vi "SDCP SMF Rx Logger - Base (version 1.1).vi"() -> ()   [LabVIEW 2020]
uses:
  Typedefs/SDCP - Serial Port Control - Commands.ctl
  Typedefs/SDCP SMF logger - SMF with timestamp.ctl
panel:
  out "error out":errorcluster
  in  "error in (no error)":errorcluster
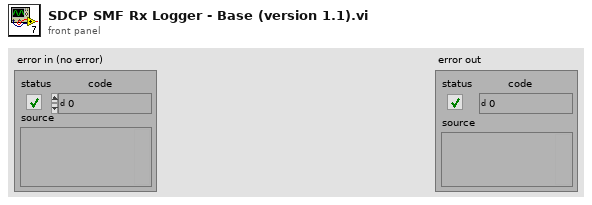
[diagram p1: front panel]
types:
  T1 = enum16{"Initialize", "Read", "Write", "Deinitialize"}
  T2 = typedef "SDCP SMF logger - SMF with timestamp.ctl" = cluster{"Bytes":u8[], "Checksum":bool, "Time (ms)":u32, "Tx/Rx":string}
  T3 = typedef "SDCP - Serial Port Control - Commands.ctl" = enum16{"Open", "Read", "Write", "Get instance", "Close"}
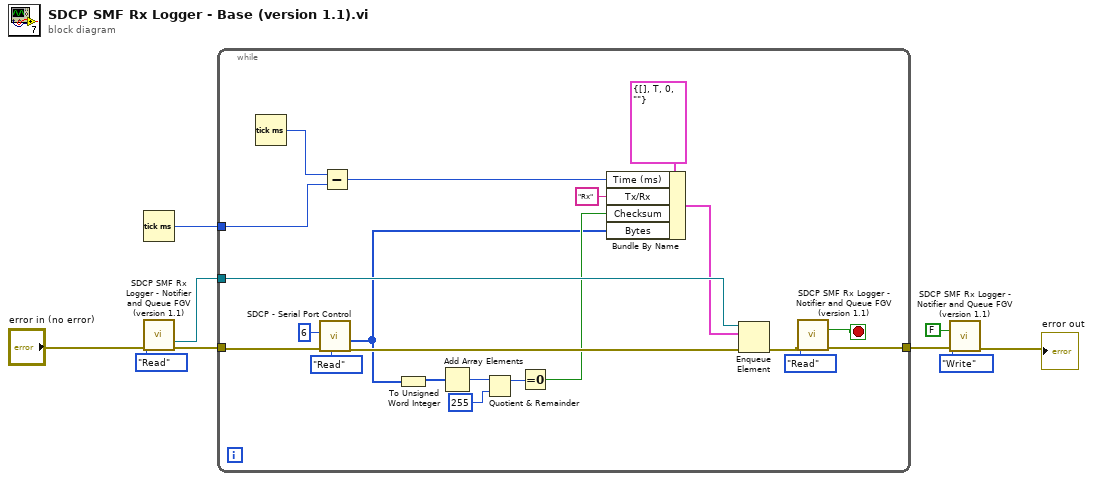
[diagram p0: block diagram]
diagram:
  n1 = Tick Count (ms)() -> (millisecond timer value=w5:u32)
  n2 = call "SDCP SMF Rx Logger - Notifier and Queue FGV (version 1.1).vi"("Commands"=T1."Read", "error in (no error)"="error in (no error)") -> ("Queue out"=w7:refnum<queue>, "error out"=w6:errorcluster)  [unwired: 9 in, 3 out]
  n3 = while {
    tunnel: w7 -> [w26]
    tunnel: w6 -> [w30]
    tunnel: w5 -> [w24]
    tunnel: [w11] -> w3
    stop <- w12 stop-if-true
    n4 = Tick Count (ms)() -> (millisecond timer value=w25:u32)
    n5 = call "SDCP - Serial Port Control.vi"("Command"=SDCP_-_Serial_Port_Control_-_Commands."Read", "error in (no error)"=w30, "Read byte count"=u32 6) -> ("error out"=w27:errorcluster, "Received bytes"=w16:u8[])  [unwired: 7 in]
    n6 = Subtract(x=w25, y=w24) -> (x-y=w22:u32)
    n7 = To Unsigned Word Integer(number=w16) -> (unsigned 16bit integer=w20:u16[])
    n8 = Add Array Elements(numeric array=w20) -> (sum=w19:u16)
    n9 = Quotient & Remainder(x=w19, y=u16 255) -> (x-y*floor(x/y)=w18:u16)  [unwired: 1 out]
    n10 = Equal To 0?(x=w18) -> (x = 0?=w17:bool)
    n11 = Bundle By Name(cluster=T2 {"Bytes"=[], "Checksum"=TRUE, "Time (ms)"=0, "Tx/Rx"=""} ("element"), "Time (ms)"=w22, "Tx/Rx"="Rx", "Checksum"=w17, "Bytes"=w16) -> (w15:T2)
    n12 = Enqueue Element(queue=w26, element=w15, error in (no error)=w27) -> (error out=w14:errorcluster)  [unwired: 1 in, 2 out]
    n13 = call "SDCP SMF Rx Logger - Notifier and Queue FGV (version 1.1).vi"("Commands"=T1."Read", "error in (no error)"=w14) -> ("Notifier value output"=w12:bool, "error out"=w11:errorcluster)  [unwired: 9 in, 3 out]
  }
  n14 = call "SDCP SMF Rx Logger - Notifier and Queue FGV (version 1.1).vi"("Commands"=T1."Write", "Notification value in"=FALSE, "error in (no error)"=w3) -> ("error out"=→"error out":errorcluster)  [unwired: 8 in, 4 out]
